vi "Toggle.vi"(11 "Boolean":bool=TRUE) -> (3 "Toggled":bool=TRUE)   [LabVIEW 2013]
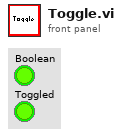
[diagram p1: front panel]
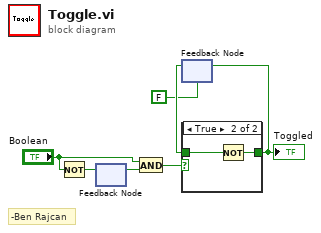
[diagram p0: block diagram]
diagram:
  # "-Ben Rajcan"
  n1 = Not(x="Boolean") -> (.not. x?=w4:bool)
  n2 = feedback #1() -> (w3:bool)  [unwired: 1 out]
  n3 = feedback-in #1(w4) -> ()
  n4 = And(x="Boolean", y=w3) -> (x .and. y?=w7:bool)
  n5 = feedback #2(FALSE) -> (w6:bool)
  n6 = case shown="True" w7 {
    tunnel: [w8 w9] -> w2
    tunnel: w6 -> [w8 w10]
    frame False {
    }
    frame True {
      n7 = Not(x=w10) -> (.not. x?=w9:bool)
    }
  }
  "Toggled" <- w2
  n8 = feedback-in #2(w2) -> ()
